vi "filter_wheel_control.vi"() -> ()   [LabVIEW 2012]
uses:
  C:/Program Files (x86)/Optec/HSFW/Custom Driver Tools/OptecHID_FilterWheelAPI.dll
  Program Files (x86)/Optec/HSFW/Custom Driver Tools/OptecHID_FilterWheelAPI.dll
panel:
  in  "Set Filter Name":string
  in  "Filter Number":i32
  in  "WheelID":i32
  in  "Name Filter Wheel":string
  out "Name":string
  out "IsAttached":bool
  out "Number of Filters":i32
  out "Centering Offset":i32
  out "IsHomed":bool
  out "WheelID":i32
  in  "Filter Wheel Position - Control":i32
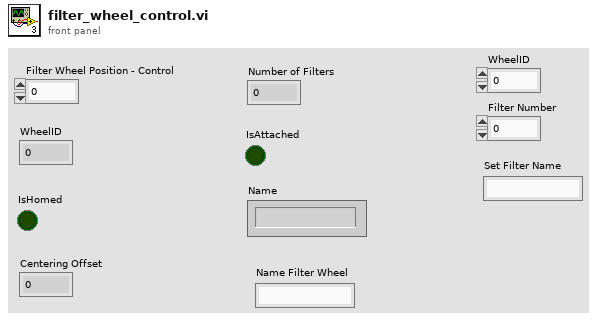
[diagram p1: front panel]
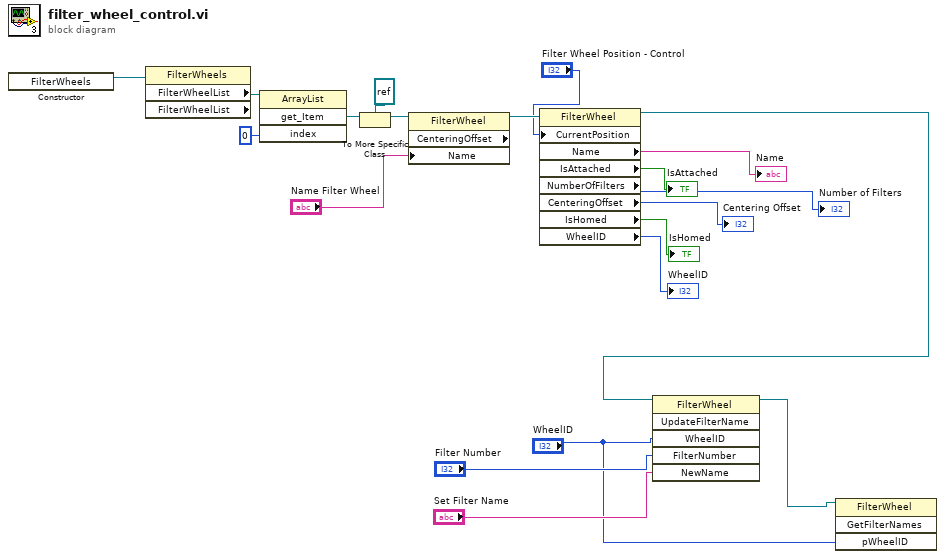
[diagram p0: block diagram]
diagram:
  n1 = constructor class="FilterWheels"() -> (reference out=w20:refnum<k24>)  [unwired: 3 in, 2 out]
  n2 = property class="FilterWheels" props=["FilterWheelList", "FilterWheelList"](reference=w20) -> ("FilterWheelList"=w19:refnum<k24>)  [unwired: 1 in, 3 out]
  n3 = invoke class="ArrayList" method="get_Item"(reference=w19, "index"=0) -> ("get_Item"=w17:refnum<k24>)  [unwired: 2 in, 3 out]
  n4 = To More Specific Class(target class=refnum<k24> refnum, reference=w17) -> (specific class reference=w15:refnum<k24>)  [unwired: 1 in, 1 out]
  n5 = property class="FilterWheel" props=["CenteringOffset", "Name"](reference=w15, "Name"="Name Filter Wheel") -> (reference out=w14:refnum<k24>)  [unwired: 1 in, 2 out]
  n6 = property class="FilterWheel"(reference=w14, "CurrentPosition"="Filter Wheel Position - Control") -> (reference out=w5:refnum<k24>, "Name"=→"Name":string, "IsAttached"=→"IsAttached":bool, "NumberOfFilters"=→"Number of Filters":i16, "CenteringOffset"=→"Centering Offset":i16, "IsHomed"=→"IsHomed":bool, "WheelID"=→"WheelID":u16)  [unwired: 1 in, 1 out]
  n7 = invoke class="FilterWheel" method="UpdateFilterName"(reference=w5, "WheelID"="WheelID", "FilterNumber"="Filter Number", "NewName"="Set Filter Name") -> (reference out=w2:refnum<k24>)  [unwired: 2 in, 5 out]
  n8 = invoke class="FilterWheel" method="GetFilterNames"(reference=w2, "pWheelID"="WheelID") -> ()  [unwired: 2 in, 4 out]
